vi "Perform_Math.vi"(0 "Input_1":dbl format="%#_13g", 5 "Input_2":dbl format="%#_13g", 13 "Operation":T1=enum."Div") -> (4 "Output":dbl)   [LabVIEW 2023]
uses:
  Controls/Operation.ctl
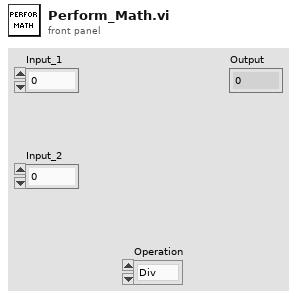
[diagram p1: front panel]
types:
  T1 = typedef "Operation.ctl" = enum16{"Add", "Sub", "Mul", "Div"}
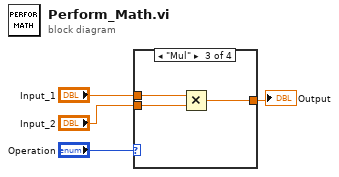
[diagram p0: block diagram]
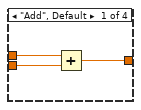
[diagram p2: hidden frame]
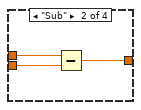
[diagram p3: hidden frame]
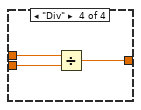
[diagram p4: hidden frame]
diagram:
  n1 = case shown="\"Mul\"" "Operation" {
    tunnel: "Input_1" -> [w7 w10 w13 w16]
    tunnel: "Input_2" -> [w6 w9 w12 w15]
    tunnel: [w5 w8 w11 w14] -> w1
    frame "Add", Default {
      n2 = Add(x=w7, y=w6) -> (x+y=w5:dbl)
    }
    frame "Sub" {
      n3 = Subtract(x=w10, y=w9) -> (x-y=w8:dbl)
    }
    frame "Mul" {
      n4 = Multiply(x=w13, y=w12) -> (x*y=w11:dbl)
    }
    frame "Div" {
      n5 = Divide(x=w16, y=w15) -> (x/y=w14:dbl)
    }
  }
  "Output" <- w1
